vi "Tolerance_Check_Fixed.vi"(9 "Value to check":dbl, 10 "Setpoint":dbl, 11 "Tolerance (+-)":dbl=1.0) -> (3 "In Range":bool)   [LabVIEW 2013]
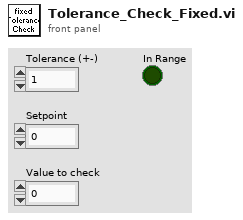
[diagram p1: front panel]
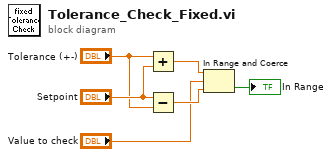
[diagram p0: block diagram]
diagram:
  n1 = Add(x="Tolerance (+-)", y="Setpoint") -> (x+y=w3:dbl)
  n2 = Subtract(x="Setpoint", y="Tolerance (+-)") -> (x-y=w4:dbl)
  n3 = In Range and Coerce(upper limit=w3, x="Value to check", lower limit=w4) -> (In Range?=→"In Range":bool)  [unwired: 1 out]
